vi "VisitorPattern_Main.vi"() -> ()   [LabVIEW 2020]
uses:
  Laser_class/Laser.lvclass
  C:/Projects/DesignPatterns/VisitorPattern/Equipment_class/Equipment.lvclass
  Oven_class/Oven.lvclass
  PrintVisitor_class/PrintVisitor.lvclass
  C:/Projects/DesignPatterns/VisitorPattern/EquipmentVisitor_class/EquipmentVisitor.lvclass
  GetCostVisitor_class/GetCostVisitor.lvclass
  Rig_class/Rig.lvclass
  Equipment_class/Equipment.lvclass
panel:
  out "StringReturn":string
  in  "Numeric":i32=2
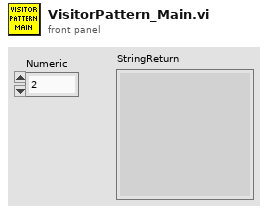
[diagram p1: front panel]
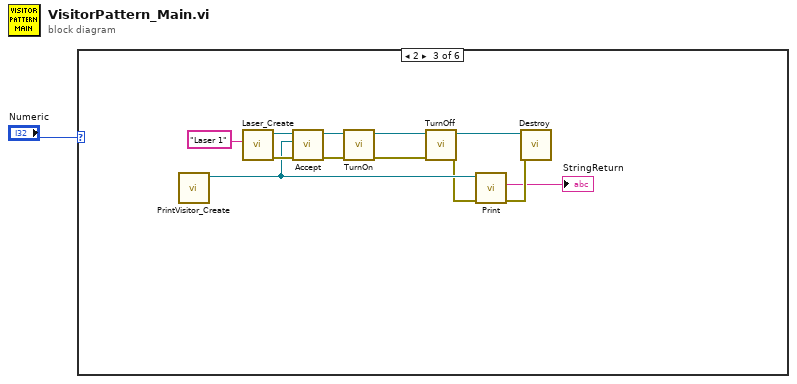
[diagram p0: block diagram]
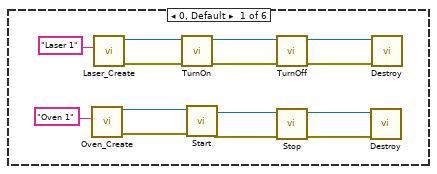
[diagram p2: hidden frame]
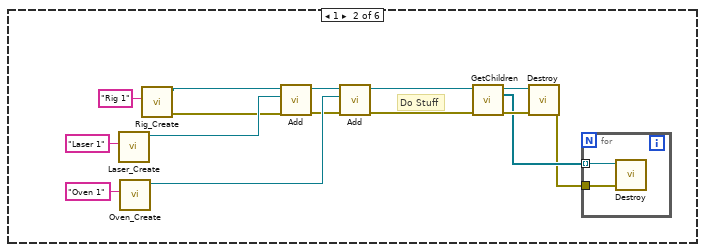
[diagram p3: hidden frame]
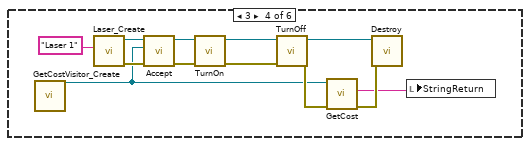
[diagram p4: hidden frame]
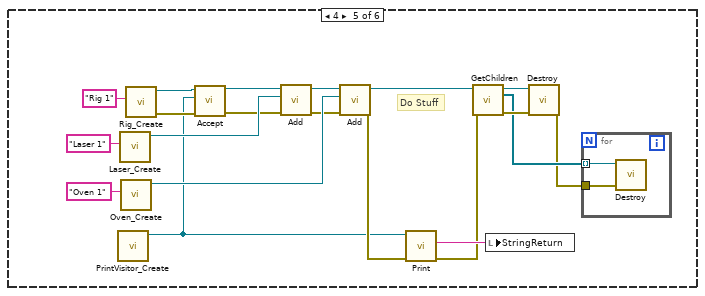
[diagram p5: hidden frame]
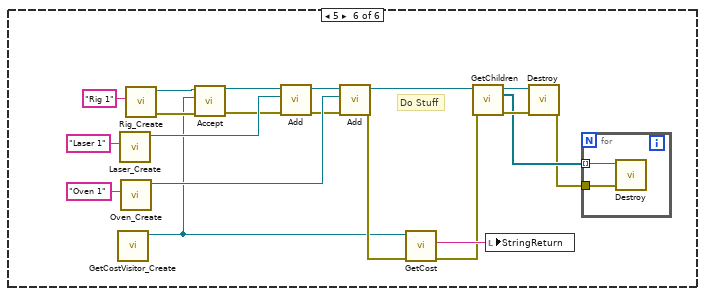
[diagram p6: hidden frame]
diagram:
  n1 = case shown="2" "Numeric" {
    frame 0, Default {
      n2 = call "Oven_Create.vi"("ID"="Oven 1") -> ("error out"=w9:errorcluster, "reference out"=w8:refnum<class "Oven.lvclass">)  [unwired: 9 in]
      n3 = call "Laser_Create.vi"("ID"="Laser 1") -> ("error out"=w15:errorcluster, "reference out"=w14:refnum<class "Laser.lvclass">)  [unwired: 9 in]
      n4 = call-dynamic "TurnOn.vi"("error in (no error)"=w15, "reference in"=w14) -> ("error out"=w13:errorcluster, "reference in"=w12:refnum<class "Laser.lvclass">)  [unwired: 8 in]
      n5 = call-dynamic "Start.vi"("error in (no error)"=w9, "reference in"=w8) -> ("error out"=w7:errorcluster, "reference in"=w6:refnum<class "Oven.lvclass">)  [unwired: 8 in]
      n6 = call-dynamic "TurnOff.vi"("error in (no error)"=w13, "reference in"=w12) -> ("error out"=w11:errorcluster, "reference in"=w10:refnum<class "Laser.lvclass">)  [unwired: 8 in]
      n7 = call-dynamic "Stop.vi"("error in (no error)"=w7, "reference in"=w6) -> ("error out"=w5:errorcluster, "reference in"=w4:refnum<class "Oven.lvclass">)  [unwired: 8 in]
      n8 = call-dynamic "Destroy.vi"("error in (no error)"=w5, "reference in"=w4) -> ()  [unwired: 8 in, 2 out]
      n9 = call-dynamic "Destroy.vi"("error in (no error)"=w11, "reference in"=w10) -> ()  [unwired: 8 in, 2 out]
    }
    frame 1 {
      # "Do Stuff"
      n10 = call "Laser_Create.vi"("ID"="Laser 1") -> ("reference out"=w26:refnum<class "Laser.lvclass">)  [unwired: 9 in, 1 out]
      n11 = call "Oven_Create.vi"("ID"="Oven 1") -> ("reference out"=w27:refnum<class "Oven.lvclass">)  [unwired: 9 in, 1 out]
      n12 = call "Rig_Create.vi"("ID"="Rig 1") -> ("error out"=w16:errorcluster, "reference out"=w17:refnum<class "Rig.lvclass">)  [unwired: 9 in]
      n13 = call-dynamic "Add.vi"("error in (no error)"=w16, "Equipment"=w26, "reference in"=w17) -> ("error out"=w24:errorcluster, "reference in"=w25:refnum<class "Rig.lvclass">)  [unwired: 7 in]
      n14 = call-dynamic "Add.vi"("error in (no error)"=w24, "Equipment"=w27, "reference in"=w25) -> ("error out"=w23:errorcluster, "reference in"=w22:refnum<class "Rig.lvclass">)  [unwired: 7 in]
      n15 = call-dynamic "GetChildren.vi"("error in (no error)"=w23, "reference in"=w22) -> ("error out"=w21:errorcluster, "Children"=w19:refnum<class "Equipment.lvclass">[], "reference in"=w20:refnum<class "Rig.lvclass">)  [unwired: 7 in]
      n16 = call-dynamic "Destroy.vi"("error in (no error)"=w21, "reference in"=w20) -> ("error out"=w18:errorcluster)  [unwired: 8 in, 1 out]
      n17 = for {
        tunnel: w19 -> [w32] mode=indexing
        tunnel: w18 -> [w31]
        n18 = call-dynamic "Destroy.vi"("error in (no error)"=w31, "reference in"=w32) -> ()  [unwired: 8 in, 2 out]
      }
    }
    frame 2 {
      n19 = call "PrintVisitor_Create.vi"() -> ("reference out"=w36:refnum<class "PrintVisitor.lvclass">)  [unwired: 10 in, 1 out]
      n20 = call "Laser_Create.vi"("ID"="Laser 1") -> ("error out"=w40:errorcluster, "reference out"=w39:refnum<class "Laser.lvclass">)  [unwired: 9 in]
      n21 = call-dynamic "Accept.vi"("error in (no error)"=w40, "EquipmentVisitor"=w36, "reference in"=w39) -> ("error out"=w37:errorcluster, "reference out"=w38:refnum<class "Laser.lvclass">)  [unwired: 7 in]
      n22 = call-dynamic "TurnOn.vi"("error in (no error)"=w37, "reference in"=w38) -> ("error out"=w44:errorcluster, "reference in"=w43:refnum<class "Laser.lvclass">)  [unwired: 8 in]
      n23 = call-dynamic "TurnOff.vi"("error in (no error)"=w44, "reference in"=w43) -> ("error out"=w35:errorcluster, "reference in"=w42:refnum<class "Laser.lvclass">)  [unwired: 8 in]
      n24 = call-dynamic "Print.vi"("error in (no error)"=w35, "reference in"=w36) -> ("error out"=w34:errorcluster, "Id String"=→"StringReturn":string)  [unwired: 7 in, 1 out]
      n25 = call-dynamic "Destroy.vi"("error in (no error)"=w34, "reference in"=w42) -> ()  [unwired: 8 in, 2 out]
    }
    frame 3 {
      n26 = call "GetCostVisitor_Create.vi"() -> ("reference out"=w46:refnum<class "GetCostVisitor.lvclass">)  [unwired: 10 in, 1 out]
      n27 = call "Laser_Create.vi"("ID"="Laser 1") -> ("error out"=w52:errorcluster, "reference out"=w51:refnum<class "Laser.lvclass">)  [unwired: 9 in]
      n28 = call-dynamic "Accept.vi"("error in (no error)"=w52, "EquipmentVisitor"=w46, "reference in"=w51) -> ("error out"=w49:errorcluster, "reference out"=w50:refnum<class "Laser.lvclass">)  [unwired: 7 in]
      n29 = call-dynamic "TurnOn.vi"("error in (no error)"=w49, "reference in"=w50) -> ("error out"=w56:errorcluster, "reference in"=w55:refnum<class "Laser.lvclass">)  [unwired: 8 in]
      n30 = call-dynamic "TurnOff.vi"("error in (no error)"=w56, "reference in"=w55) -> ("error out"=w48:errorcluster, "reference in"=w54:refnum<class "Laser.lvclass">)  [unwired: 8 in]
      n31 = call-dynamic "GetCost.vi"("error in (no error)"=w48, "reference in"=w46) -> ("error out"=w47:errorcluster, "Cost String"=w45:string)  [unwired: 7 in, 1 out]
      n32 = call-dynamic "Destroy.vi"("error in (no error)"=w47, "reference in"=w54) -> ()  [unwired: 8 in, 2 out]
      n33 = local write "StringReturn"(w45) -> ()
    }
    frame 4 {
      # "Do Stuff"
      n34 = call "PrintVisitor_Create.vi"() -> ("reference out"=w57:refnum<class "PrintVisitor.lvclass">)  [unwired: 10 in, 1 out]
      n35 = call "Laser_Create.vi"("ID"="Laser 1") -> ("reference out"=w72:refnum<class "Laser.lvclass">)  [unwired: 9 in, 1 out]
      n36 = call "Oven_Create.vi"("ID"="Oven 1") -> ("reference out"=w73:refnum<class "Oven.lvclass">)  [unwired: 9 in, 1 out]
      n37 = call "Rig_Create.vi"("ID"="Rig 1") -> ("error out"=w63:errorcluster, "reference out"=w64:refnum<class "Rig.lvclass">)  [unwired: 9 in]
      n38 = call-dynamic "Accept.vi"("error in (no error)"=w63, "EquipmentVisitor"=w57, "reference in"=w64) -> ("error out"=w61:errorcluster, "reference in"=w62:refnum<class "Rig.lvclass">)  [unwired: 7 in]
      n39 = call-dynamic "Add.vi"("error in (no error)"=w61, "Equipment"=w72, "reference in"=w62) -> ("error out"=w70:errorcluster, "reference in"=w71:refnum<class "Rig.lvclass">)  [unwired: 7 in]
      n40 = call-dynamic "Add.vi"("error in (no error)"=w70, "Equipment"=w73, "reference in"=w71) -> ("error out"=w59:errorcluster, "reference in"=w69:refnum<class "Rig.lvclass">)  [unwired: 7 in]
      n41 = call-dynamic "Print.vi"("error in (no error)"=w59, "reference in"=w57) -> ("error out"=w58:errorcluster, "Id String"=w60:string)  [unwired: 7 in, 1 out]
      n42 = call-dynamic "GetChildren.vi"("error in (no error)"=w58, "reference in"=w69) -> ("error out"=w68:errorcluster, "Children"=w66:refnum<class "Equipment.lvclass">[], "reference in"=w67:refnum<class "Rig.lvclass">)  [unwired: 7 in]
      n43 = local write "StringReturn"(w60) -> ()
      n44 = call-dynamic "Destroy.vi"("error in (no error)"=w68, "reference in"=w67) -> ("error out"=w65:errorcluster)  [unwired: 8 in, 1 out]
      n45 = for {
        tunnel: w66 -> [w78] mode=indexing
        tunnel: w65 -> [w77]
        n46 = call-dynamic "Destroy.vi"("error in (no error)"=w77, "reference in"=w78) -> ()  [unwired: 8 in, 2 out]
      }
    }
    frame 5 {
      # "Do Stuff"
      n47 = call "GetCostVisitor_Create.vi"() -> ("reference out"=w79:refnum<class "GetCostVisitor.lvclass">)  [unwired: 10 in, 1 out]
      n48 = call "Laser_Create.vi"("ID"="Laser 1") -> ("reference out"=w94:refnum<class "Laser.lvclass">)  [unwired: 9 in, 1 out]
      n49 = call "Oven_Create.vi"("ID"="Oven 1") -> ("reference out"=w95:refnum<class "Oven.lvclass">)  [unwired: 9 in, 1 out]
      n50 = call "Rig_Create.vi"("ID"="Rig 1") -> ("error out"=w85:errorcluster, "reference out"=w86:refnum<class "Rig.lvclass">)  [unwired: 9 in]
      n51 = call-dynamic "Accept.vi"("error in (no error)"=w85, "EquipmentVisitor"=w79, "reference in"=w86) -> ("error out"=w83:errorcluster, "reference in"=w84:refnum<class "Rig.lvclass">)  [unwired: 7 in]
      n52 = call-dynamic "Add.vi"("error in (no error)"=w83, "Equipment"=w94, "reference in"=w84) -> ("error out"=w92:errorcluster, "reference in"=w93:refnum<class "Rig.lvclass">)  [unwired: 7 in]
      n53 = call-dynamic "Add.vi"("error in (no error)"=w92, "Equipment"=w95, "reference in"=w93) -> ("error out"=w81:errorcluster, "reference in"=w91:refnum<class "Rig.lvclass">)  [unwired: 7 in]
      n54 = call-dynamic "GetCost.vi"("error in (no error)"=w81, "reference in"=w79) -> ("error out"=w80:errorcluster, "Cost String"=w82:string)  [unwired: 7 in, 1 out]
      n55 = call-dynamic "GetChildren.vi"("error in (no error)"=w80, "reference in"=w91) -> ("error out"=w90:errorcluster, "Children"=w88:refnum<class "Equipment.lvclass">[], "reference in"=w89:refnum<class "Rig.lvclass">)  [unwired: 7 in]
      n56 = local write "StringReturn"(w82) -> ()
      n57 = call-dynamic "Destroy.vi"("error in (no error)"=w90, "reference in"=w89) -> ("error out"=w87:errorcluster)  [unwired: 8 in, 1 out]
      n58 = for {
        tunnel: w88 -> [w100] mode=indexing
        tunnel: w87 -> [w99]
        n59 = call-dynamic "Destroy.vi"("error in (no error)"=w99, "reference in"=w100) -> ()  [unwired: 8 in, 2 out]
      }
    }
  }
